vi "MorphStructuringElementCore.vi"(5 "Shape":T2, 7 "Anchor (Default: -1, -1 Use Centre)":T3={"x"=-1, "y"=-1}, 8 "error in (no error)":errorcluster, 11 "Size":T1) -> (0 "error out":errorcluster, 3 "Structuring Element":bool[][](array[boolean]))   [LabVIEW 2020, in "g_ar_toolkit.image.lvlib"]
uses:
  g_ar_toolkit.image.lvlib
  g_ar_toolkit.common/Image Point (Integer).ctl
  MorphologyStructuredElementShape.ctl
  g_ar_toolkit.common/Image Size (Integer).ctl
  g_ar_toolkit.common/g_ar_toolkit.common.lvlib
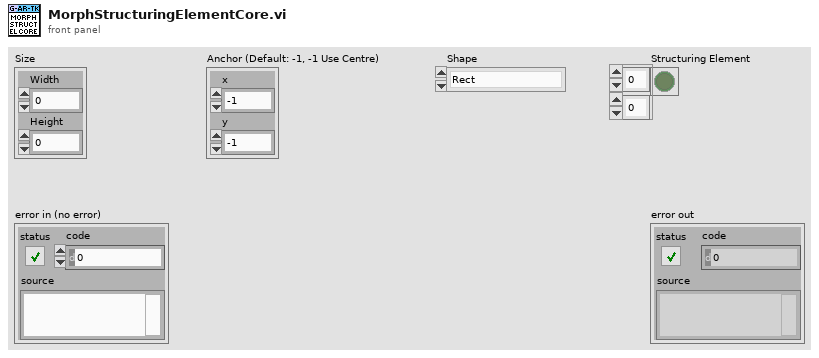
[diagram p1: front panel]
types:
  T1 = typedef "g_ar_toolkit.common.lvlib/Image Size (Integer).ctl" = cluster{"Width":u16, "Height":u16}
  T2 = typedef "g_ar_toolkit.image.lvlib/MorphologyStructuredElementShape.ctl" = enum16{"Rect", "Cross", "Elipse"}
  T3 = typedef "g_ar_toolkit.common.lvlib/Image Point (Integer).ctl" = cluster{"x":i32, "y":i32}
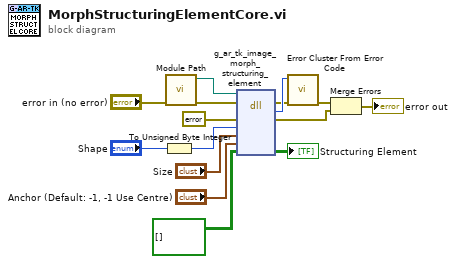
[diagram p0: block diagram]
diagram:
  n1 = To Unsigned Byte Integer(number="Shape") -> (unsigned 8bit integer=w1:u8)
  n2 = call "Module Path.vi"("error in (no error)"="error in (no error)") -> ("error out"=w9:errorcluster, "Path"=w10:path)  [unwired: 9 in]
  n3 = dll-call lib="?" fn="g_ar_tk_image_morph_structuring_element" ("g_ar_toolkit.*.*:g_ar_tk_image_get_text_size")(path in=w10, error in=w9, "error_cluster"=errorcluster {"status"=FALSE, "code"=0, "source"=""} ("error constant"), "shape"=w1, "size"="Size", "anchor"="Anchor (Default: -1, -1 Use Centre)", "structuring_element"=bool[][] [] ("Array")) -> (error out=w4:errorcluster, "MgErr"=w5:i32, "error_cluster"=w8:errorcluster, "structuring_element"=→"Structuring Element":bool[][])  [unwired: 4 in, 1 out]
  n4 = call <vilib>:"Error Cluster From Error Code.vi"("error in (no error)"=w4, "error code (0)"=w5) -> ("error out"=w6:errorcluster)  [unwired: 7 in]
  n5 = Merge Errors(w6, w8) -> (→"error out":errorcluster)
